vi "Instantiate.vi"(0 "LV MDI.lvclass":refnum<class "LV MDI.lvclass">, 5 "PathIn":path, 11 "Error in":errorcluster) -> (4 "LV MDI.lvclass":refnum<class "LV MDI.lvclass">, 8 "Path Out":path, 15 "Error Out":errorcluster)   [LabVIEW 2016, in "LV MDI.lvclass"]
uses:
  LV MDI.lvclass
  Document/Document.lvclass
  Document/Child Classes/LV Doc/LV Doc.lvclass
  Document/Child Classes/Py Doc/Py Doc.lvclass
  LV MDI.lvclass/LV MDI.ctl
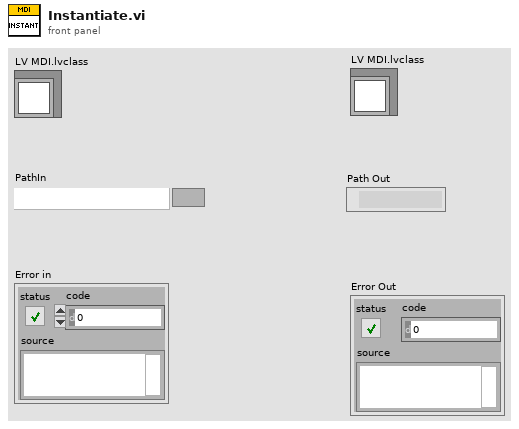
[diagram p1: front panel]
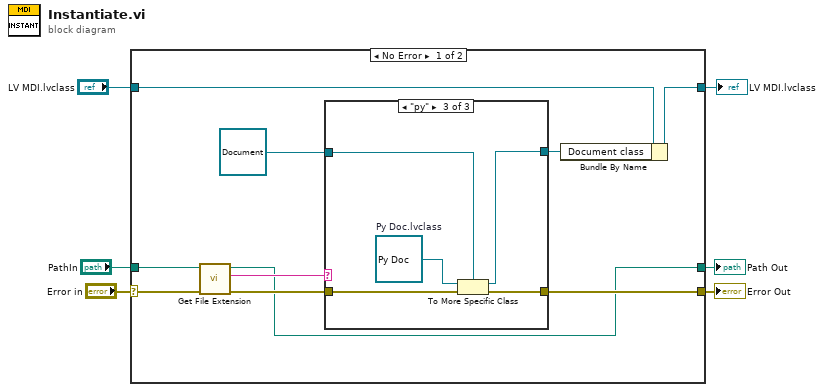
[diagram p0: block diagram]
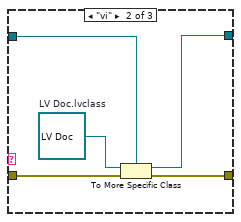
[diagram p3: hidden frame]
diagram:
  n1 = case shown="No Error" "Error in" {
    selector: "Error in" -> [w16 w31]
    tunnel: [w14 w31] -> w5
    tunnel: "PathIn" -> [w12 w29]
    tunnel: "LV MDI.lvclass" -> [w10 w30]
    tunnel: [w9 w30] -> w2
    tunnel: [w7 w29] -> w1
    frame No Error {
      n2 = call <vilib>:"Get File Extension.vi"("error in (no error)"=w16, "file"=w12) -> ("error out"=w15:errorcluster, "lowercase file extension"=w13:string, "dup file"=w7:path)  [unwired: 5 in, 2 out]
      n3 = case shown="\"py\"" w13 {
        tunnel: w15 -> [w18 w23 w28]
        tunnel: [w18 w22 w27] -> w14
        tunnel: refnum<class "Document.lvclass"> refnum ("Document.lvclass") -> [w17 w20 w25]
        tunnel: [w17 w19 w24] -> w8
        frame Default {
        }
        frame "vi" {
          w21 = refnum<class "LV Doc.lvclass"> refnum  # LV Doc.lvclass
          n4 = To More Specific Class(target class=w20, reference=w21, error in=w23) -> (specific class reference=w19:refnum<class "Document.lvclass">, error out=w22:errorcluster)
        }
        frame "py" {
          w26 = refnum<class "Py Doc.lvclass"> refnum  # Py Doc.lvclass
          n5 = To More Specific Class(target class=w25, reference=w26, error in=w28) -> (specific class reference=w24:refnum<class "Document.lvclass">, error out=w27:errorcluster)
        }
      }
      n6 = Bundle By Name(cluster=w10, "Document class"=w8) -> (w9:refnum<class "LV MDI.lvclass">)
    }
    frame Error {
    }
  }
  "Error Out" <- w5
  "LV MDI.lvclass" <- w2
  "Path Out" <- w1
